vi "ROI_to_norm_ROI_Convertor.vi"(10 "Experiment folder path":path, 11 "XYZ Coordinates":T1[](array[typedef]) {"Apparent Frame Size" format="%#_6f"; "Original FOV (um)" format="%#_6f"; "Pixels per miniscan" format="%#_6f"; "Dwell Time per pixel" format="%#_6f"; "Resolution" format="%#_6f"; "ROI group ID" format="%#_6f"; "Laser Power (%)" format="%#_6f"; "Zoom" format="%#_6f"; "Frame Size" format="%#_6f"; "Number of lines" format="%#_6f"; "Composite ID" format="%#_6f"; "Angle (deg)" format="%#_6f"; "ROI Time (ns)" format="%#_6f"; "ROI ID" format="%#_6f"; "Pixels in ROI" format="%#_6f"; "ROI index" format="%#_6f"; "Z stop" format="%#_6f"; "Y stop" format="%#_6f"; "X stop" format="%#_6f"; "Z start" format="%#_6f"; "X start" format="%#_6f"; "Y start" format="%#_6f"}) -> (3 "norm_XYZ_Coordinates":T1[](array[typedef]) {"Apparent Frame Size" format="%#_6f"; "Original FOV (um)" format="%#_6f"; "Pixels per miniscan" format="%#_6f"; "Dwell Time per pixel" format="%#_6f"; "Resolution" format="%#_6f"; "ROI group ID" format="%#_6f"; "Laser Power (%)" format="%#_6f"; "Zoom" format="%#_6f"; "Frame Size" format="%#_6f"; "Number of lines" format="%#_6f"; "Composite ID" format="%#_6f"; "Angle (deg)" format="%#_6f"; "ROI Time (ns)" format="%#_6f"; "ROI ID" format="%#_6f"; "Pixels in ROI" format="%#_6f"; "ROI index" format="%#_6f"; "Z stop" format="%#_6f"; "Y stop" format="%#_6f"; "X stop" format="%#_6f"; "Z start" format="%#_6f"; "X start" format="%#_6f"; "Y start" format="%#_6f"})   [LabVIEW 2020]
uses:
  Visualisation/Functional Imaging Viewer/Typedefs/ROI parameters data type.ctl
  Global Variables/gl_UI Ctrl Refs.vi
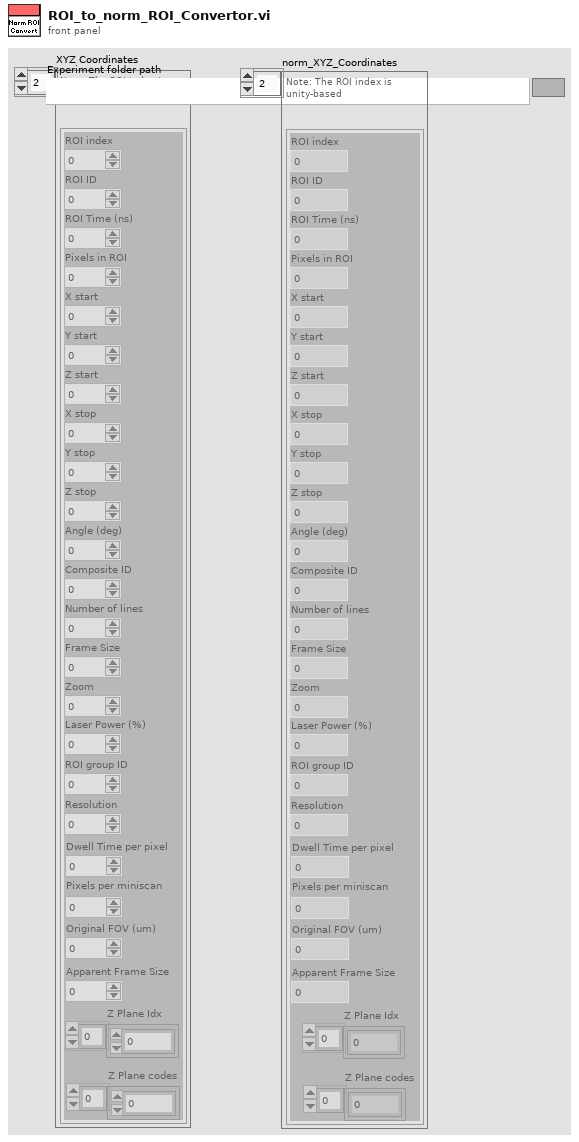
[diagram p1: front panel]
types:
  T1 = typedef "ROI parameters data type.ctl" = cluster{"ROI index":dbl, "ROI ID":dbl, "ROI Time (ns)":dbl, "Pixels in ROI":dbl, "X start":dbl, "Y start":dbl, "Z start":dbl, "X stop":dbl, "Y stop":dbl, "Z stop":dbl, "Angle (deg)":dbl, "Composite ID":dbl, "Number of lines":dbl, "Frame Size":dbl, "Zoom":dbl, "Laser Power (%)":dbl, "ROI group ID":dbl, "Resolution":dbl, "Dwell Time per pixel":dbl, "Pixels per miniscan":dbl, "Original FOV (um)":dbl, "Apparent Frame Size":dbl, "Z Plane Idx":i32[], "Z Plane codes":i32[]}
  T2 = typedef "Image Type" = u32
  T3 = typedef "UI ctrl refs cluster.ctl" = cluster{"Top level VI path":path, "Top level VI ref":refnum<vi>, "User menu ref":refnum<k9>, "Sub Panel control":refnum<vi>, "Imaging Param Tab":refnum<vi>, "Occurrence-Start drivers":refnum<k4>, "Occurrence-Speed logging initialised":refnum<k4>, "Occurrence-XYZ stage initialised":refnum<k4>, "Exit button":refnum<vi>, "Status ind":refnum<vi>, "Set as origin":refnum<vi>, "Speed Logging":refnum<vi>, "Time Lapse":refnum<vi>, "Live Imaging":refnum<vi>, "AOL Z Stack":refnum<vi>, "Motor Z Stack":refnum<vi>, "Funct Acq button":refnum<vi>, "Hard Shutter":refnum<vi>, "Virtual Shutter":refnum<vi>, "Laser Power":refnum<vi>, "AOL Mode":refnum<vi>, "Frame Size":refnum<vi>, "Field of View":refnum<vi>, "Dwell Time":refnum<vi>, "Zoom":refnum<vi>, "AOL Z":refnum<vi>, "Objective":refnum<vi>, "Axis":refnum<vi>, "Paths & Names":refnum<vi>, "Experiment folder path (ind.)":refnum<vi>, "Last State (Ind.)":refnum<vi>, "Averages":refnum<vi>, "Angle (degrees)":refnum<vi>, "X centre":refnum<vi>, "Y centre":refnum<vi>, "Plane Mode":refnum<vi>, "# Planes":refnum<vi>, "Z Start":refnum<vi>, "Z Stop":refnum<vi>, "Z Step":refnum<vi>, "PMT 1":refnum<vi>, "PMT 2":refnum<vi>, "Stage XYZ Position":refnum<vi>, "Pockels@Z Start":refnum<vi>, "Pockels@Z Stop":refnum<vi>, "Obtain Z Start":refnum<vi>, "Obtain Z Stop":refnum<vi>, "Live stim.trig.period":refnum<vi>, "Live stim.trig.enable":refnum<vi>, "Movement Correction":refnum<vi>, "Load Reference Image":refnum<vi>, "XY Stage Move":refnum<vi>, "MovCor Cluster":refnum<vi>, "RefDAQParam":refnum<vi>, "Funct. Acq. Pockels Modulation":refnum<vi>, "Ref Laser Power":refnum<vi>, "Enable Video Recording":refnum<vi>, "Video Record-Live Imaging":refnum<vi>, "Video Record-Funct acq":refnum<vi>, "Reference Source":refnum<vi>, "AOL Z-stack Chirps Ready (ind)":refnum<vi>, "Target time between mov.cor. ref triggers (ms)":refnum<vi>, "Funct. Acq. Ref frame save":refnum<vi>, "Tracking button":refnum<vi>, "Show ref plots window":refnum<vi>, "Center freq ind (nm)":refnum<vi>, "Pickup mode (ind)":refnum<vi>, "Logging queue (ind)":refnum<vi>, "Back aperture power (ind.)":refnum<vi>, "Power after objective (ind.)":refnum<vi>, "Switch user":refnum<vi>, "Ls1 Conn. Status":refnum<vi>, "Ls1Tuning Status":refnum<vi>, "Ls1 Faults":refnum<vi>, "Ls1 Connection":refnum<vi>, "Ls1 Mode":refnum<vi>, "Ls1 POWER [mW]":refnum<vi>, "Ls1Shutter":refnum<vi>, "Ls1 Wavelength":refnum<vi>, "Ls1 Note":refnum<vi>, "Ls1 Confirm Wav":refnum<vi>, "Ls1 PreChrp Prism1":refnum<vi>, "Ls1 PreChrp Prism2":refnum<vi>, "Ls1 wav top Ind":refnum<vi>, "Ls1 power top Ind":refnum<vi>, "Ls1 Pump peak Hold":refnum<vi>, "Ls1 Status Ind":refnum<vi>, "Ls1 wav cancel":refnum<vi>, "Experiment Type":refnum<vi>, "Biology Information":refnum<vi>, "Camera recording status":refnum<vi>}
  T4 = typedef "Fixed strings.ctl" = cluster{"ROI file name":string, "Normalised ROI file name":string, "Zplane Pockels values file name":string, "Functional data folder name":string, "Experiment Header file name":string, "Z-stack images folder name":string, "Groups setup rel. path":string, "Groups text file rel. path":string, "TDMS files folder name (F.img)":string, "TDMS files folder name (V.acq)":string, "TDMS files folder name (Pl.acq)":string, "Cycle rel times sequence file":string, "Dynamically called VIs folder name":string, "Time Series folder base name":string}
  T5 = typedef "IMAQ Image.ctl" = refnum<image>
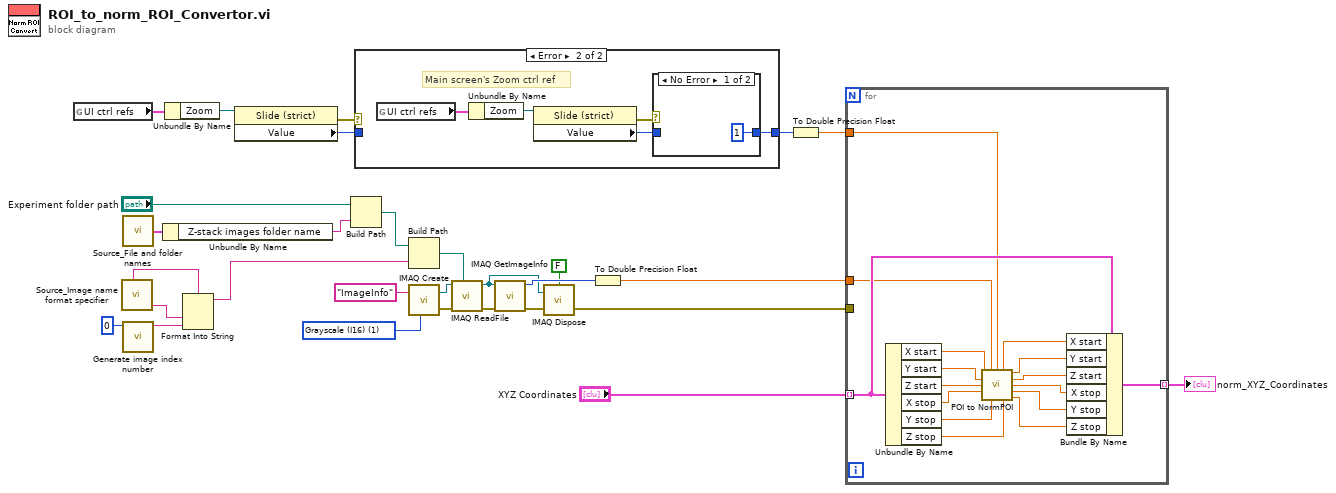
[diagram p0: block diagram]
diagram:
  w27 = T2 1 items=["Grayscale (U8)", "Grayscale (I16)", "Grayscale (SGL)", "Complex (CSG)", "RGB (U32)", "HSL (U32)", "RGB (U64)", "Grayscale (U16)"] ("Image Type")
  n1 = global read "gl_UI Ctrl Refs.vi" "UI ctrl refs"() -> (w7:T3)
  n2 = call "Source_Image name format specifier.vi"() -> ("Z-Stack Image name format specifier"=w12:string, "Green channel name"=w8:string)  [unwired: 5 in, 1 out]
  n3 = call "Source_File and folder names.vi"() -> ("Fixed strings"=w16:T4)  [unwired: 1 in]
  n4 = call "Generate image index number.vi"("FOR loop iteration or existing number of files"=0) -> ("Number in string representation (padded with zeroes)"=w10:string)  [unwired: 10 in]
  n5 = Unbundle By Name(w16) -> ("Z-stack images folder name"=w15:string)
  n6 = Unbundle By Name(w7) -> ("Zoom"=w6:refnum<vi>)
  n7 = Format Into String(format string=w12, w8, w10) -> (resulting string=w9:string)  [unwired: 2 in, 1 out]
  n8 = property class="Slide (strict)"(reference=w6) -> (error out=w4:errorcluster, "Value"=w2:i8)  [unwired: 1 in, 1 out]
  n9 = Build Path(base path="Experiment folder path", name or relative path=w15) -> (appended path=w18:path)
  n10 = case shown="Error" w4 {
    tunnel: w2 -> [w30 _]
    tunnel: [w30 w31] -> w3
    frame No Error {
    }
    frame Error {
      # "Main screen's Zoom ctrl ref"
      n11 = global read "gl_UI Ctrl Refs.vi" "UI ctrl refs"() -> (w35:T3)
      n12 = Unbundle By Name(w35) -> ("Zoom"=w34:refnum<vi>)
      n13 = property class="Slide (strict)"(reference=w34) -> (error out=w33:errorcluster, "Value"=w32:i8)  [unwired: 1 in, 1 out]
      n14 = case shown="No Error" w33 {
        tunnel: w32 -> [_ w37]
        tunnel: [i8 1 ("Value") w37] -> w31
        frame No Error {
        }
        frame Error {
        }
      }
    }
  }
  n15 = Build Path(base path=w18, name or relative path=w9) -> (appended path=w24:path)
  n16 = call "IMAQ Create"("Image Name"="ImageInfo", "Image Type"=w27) -> ("New Image"=w25:T5, "error out"=w23:errorcluster)  [unwired: 3 in]
  n17 = call "IMAQ ReadFile"("File Path"=w24, "error in (no error)"=w23, "Image"=w25) -> ("error out"=w22:errorcluster, "Image Out"=w20:T5)  [unwired: 4 in, 3 out]
  n18 = call "IMAQ GetImageInfo"("error in (no error)"=w22, "Image"=w20) -> ("error out"=w21:errorcluster, "X Resolution"=w28:i32)  [unwired: 2 in, 6 out]
  n19 = call "IMAQ Dispose"("All Images? (No)"=FALSE, "Image"=w20, "error in (no error)"=w21) -> ("error out"=w13:errorcluster)  [unwired: 3 in]
  n20 = To Double Precision Float(number=w28) -> (double precision float=w5:dbl)
  n21 = To Double Precision Float(number=w3) -> (double precision float=w1:dbl)
  n22 = for {
    tunnel: "XYZ Coordinates" -> [w40] mode=indexing
    tunnel: [w50] -> w14 mode=indexing
    tunnel: w5 -> [w39]
    tunnel: w13 -> [_]
    tunnel: w1 -> [w38]
    n23 = Unbundle By Name(w40) -> ("X start"=w53:dbl, "Y start"=w52:dbl, "Z start"=w51:dbl, "X stop"=w46:dbl, "Y stop"=w45:dbl, "Z stop"=w44:dbl)
    n24 = call "POI to NormPOI.vi"("X start"=w53, "FrameSize"=w39, "Zoom"=w38, "Y start"=w52, "Z start"=w51, "X stop"=w46, "Y stop"=w45, "Z stop"=w44) -> ("Norm XStart"=w48:dbl, "Norm YStart"=w47:dbl, "Norm ZStart"=w49:dbl, "Norm XStop"=w43:dbl, "Norm YStop"=w42:dbl, "Norm ZStop"=w41:dbl)  [unwired: 2 in]
    n25 = Bundle By Name(cluster=w40, "X start"=w48, "Y start"=w47, "Z start"=w49, "X stop"=w43, "Y stop"=w42, "Z stop"=w41) -> (w50:T1)
  }
  "norm_XYZ_Coordinates" <- w14
